vi "Use Events.vi"(8 "error in (no error)":errorcluster, 11 "DAQmxAI in":refnum<class "DAQmxAI.lvclass">) -> (0 "error out":errorcluster, 2 "Use Events":bool, 3 "DAQmxAI out":refnum<class "DAQmxAI.lvclass">)   [LabVIEW 2020, in "VolatusDAQ.lvlib" / "DAQmxAI.lvclass"]
uses:
  DAQmxAI.lvclass
  DAQmxAI.lvclass/DAQmxAI.ctl
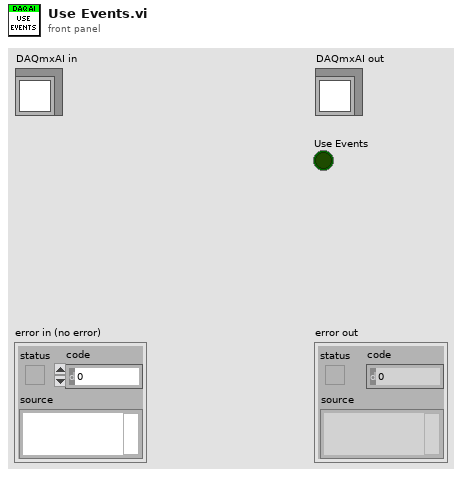
[diagram p1: front panel]
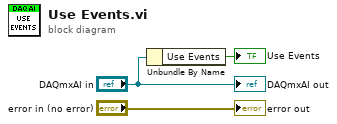
[diagram p0: block diagram]
diagram:
  n1 = Unbundle By Name("DAQmxAI in") -> ("Use Events"=→"Use Events":bool)
  "error out" <- "error in (no error)"
  "DAQmxAI out" <- "DAQmxAI in"
